vi "Shutdown.vi"(8 "error in":errorcluster, 11 "PRM in":refnum<class "PRM.lvclass">) -> (0 "error out":errorcluster, 3 "PRM out":refnum<class "PRM.lvclass">)   [LabVIEW 2019, in "PRM.lvlib" / "PRM.lvclass"]
uses:
  Library/PRM.lvclass
  builds/Instruments/Instruments.lvlibp/Library/Instruments.lvclass
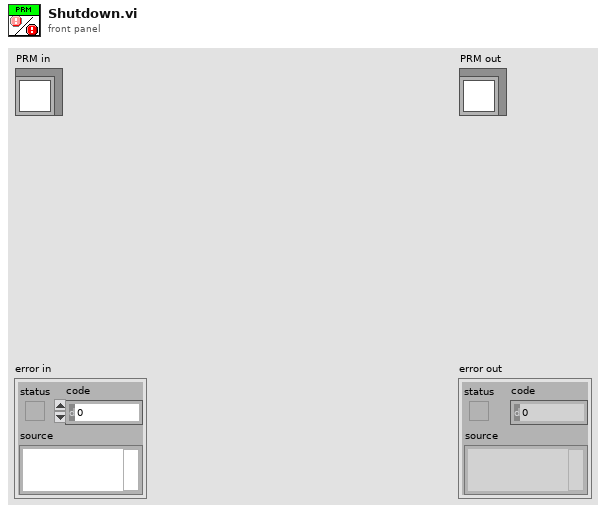
[diagram p1: front panel]
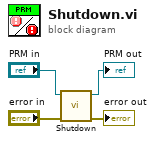
[diagram p0: block diagram]
diagram:
  n1 = call-parent "Shutdown.vi"("error in"="error in", "Instruments in"="PRM in") -> ("error out"=→"error out":errorcluster, "Instruments out"=→"PRM out":refnum<class "PRM.lvclass">)  [unwired: 8 in]
